vi "Chirp packets filename.vi"() -> (1 "concatenated string":string, 3 "Packets file path":path)   [LabVIEW 2013]
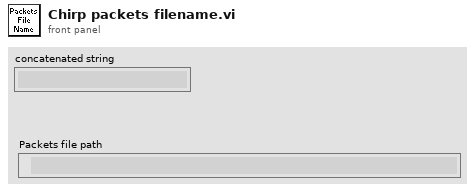
[diagram p1: front panel]
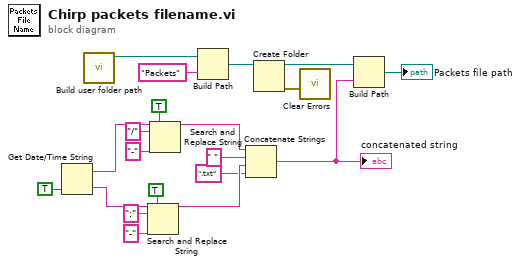
[diagram p0: block diagram]
diagram:
  n1 = Get Date/Time String(want seconds? (F)=TRUE) -> (date string=w17:string, time string=w13:string)  [unwired: 2 in]
  n2 = call "Build user folder path.vi"() -> ("Daily folder path with user folder appended?"=w1:path)  [unwired: 11 in]
  n3 = Search and Replace String(replace all?=TRUE ("replace all? (F)"), input string=w13, search string=":", replace string="-" ("replace string (\"\")")) -> (result string=w11:string)  [unwired: 4 in, 3 out]
  n4 = Search and Replace String(replace all?=TRUE ("replace all? (F)"), input string=w17, search string="/", replace string="-" ("replace string (\"\")")) -> (result string=w12:string)  [unwired: 4 in, 3 out]
  n5 = Build Path(base path=w1, name or relative path="Packets") -> (appended path=w7:path)
  n6 = Concatenate Strings(w12, " " ("string"), w11, ".txt" ("string")) -> (w4:string)
  "concatenated string" <- w4
  n7 = Create Folder(path (use dialog)=w7) -> (created path=w6:path, error out=w2:errorcluster)  [unwired: 2 in, 1 out]
  n8 = call <vilib>:"Clear Errors.vi"("error in (no error)"=w2) -> ()  [unwired: 6 in, 1 out]
  n9 = Build Path(base path=w6, name or relative path=w4) -> (appended path=→"Packets file path":path)
